vi "Invoke Specific Command.vi"(0 "LVx Command in":refnum<class "LVx.lvclass">, 5 "Session ID":string, 11 "error in (no error)":errorcluster) -> (4 "LVx Command out":refnum<class "LVx.lvclass">, 15 "error out":errorcluster)   [LabVIEW 2011, in "LVx.lvlib" / "LVx.lvclass"]
uses:
  LVx.lvclass
  LVx.lvclass/LVx.ctl
  LVx.lvlib
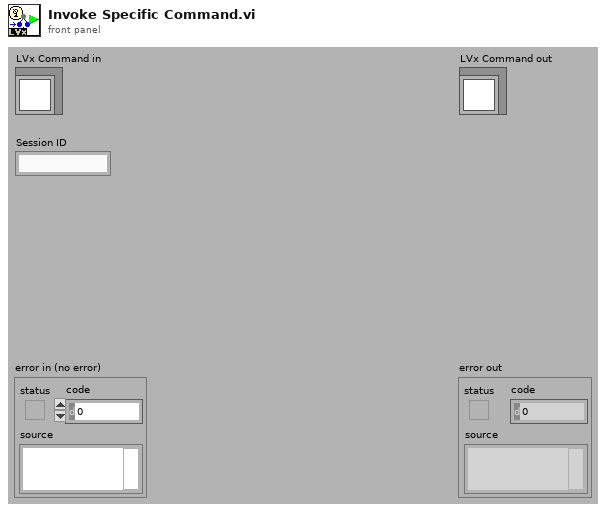
[diagram p1: front panel]
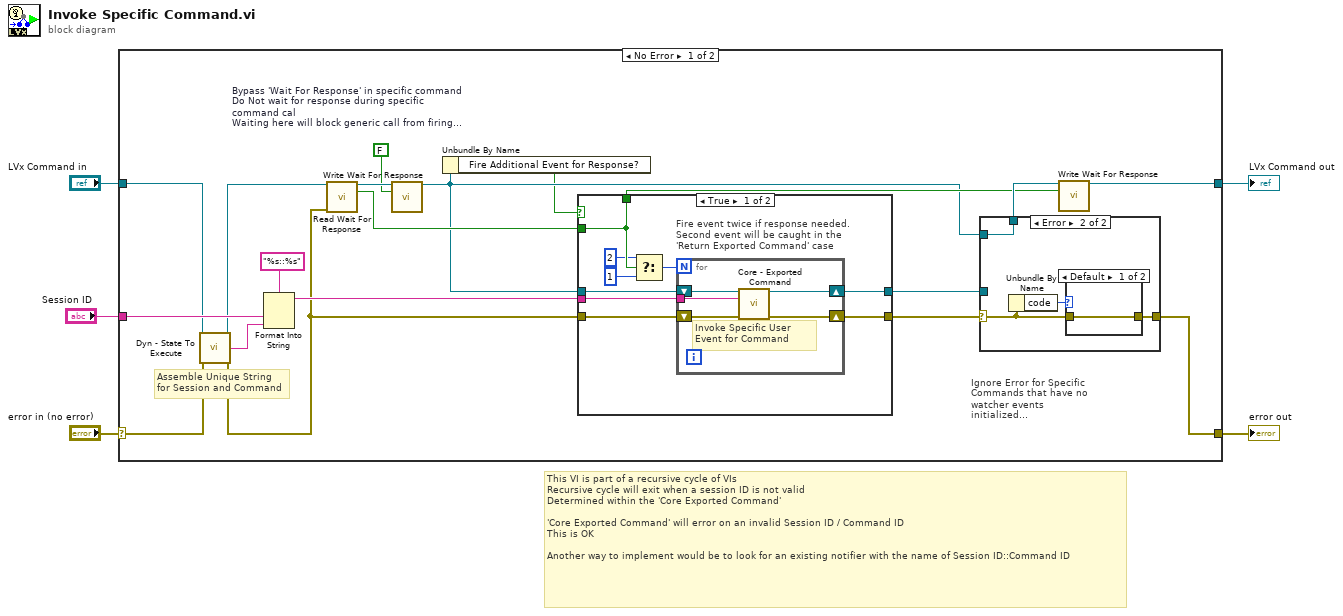
[diagram p0: block diagram]
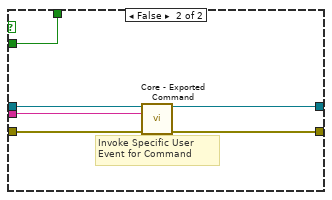
[diagram p2: hidden frame]
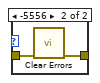
[diagram p4: hidden frame]
diagram:
  # "This VI is part of a recursive cycle of VIs\nRecursive cycle will exit when a session ID is not valid\nDetermined within the 'Core Exported Command'\n\n'Core Exported Command' will error on an invalid Session ID / Command ID\nThis is OK\n\nAnother way to implement would be to look for an existing notifier with the name of Session ID::Command ID"
  n1 = case shown="No Error" "error in (no error)" {
    selector: "error in (no error)" -> [w20 w55]
    tunnel: [w16 w55] -> w4
    tunnel: [w10 w54] -> w2
    tunnel: "LVx Command in" -> [w19 w54]
    tunnel: "Session ID" -> [w24 _]
    frame No Error {
      w12 = FALSE  # Bypass 'Wait For Response' in specific command Do Not wait for response during specific command cal Waiting here will block generic call from firing because of wait Response is caught in the calling VI (F)
      # "Assemble Unique String for Session and Command"
      n2 = call-dynamic "Dyn - State To Execute.vi"("LVx Command in"=w19, "error in (no error)"=w20) -> ("LVx Command out"=w15:refnum<class "LVx.lvclass">, "State To Execute"=w23:string, "error out"=w13:errorcluster)  [unwired: 11 in]
      n3 = Format Into String(format string="%s::%s", w24, w23) -> (resulting string=w21:string)  [unwired: 2 in, 1 out]
      n4 = call-dynamic "Read Wait For Response.vi"("LVx.lvclass in"=w15, "error in (no error)"=w13) -> ("LVx.lvclass out"=w14:refnum<class "LVx.lvclass">, "Wait For Response?"=w9:bool)  [unwired: 11 in, 1 out]
      n5 = call "Write Wait For Response.vi"("LVx.lvclass in"=w14, "Wait For Response? (T)"=w12) -> ("LVx.lvclass out"=w7:refnum<class "LVx.lvclass">)  [unwired: 12 in, 1 out]
      n6 = Unbundle By Name(w7) -> ("Fire Additional Event for Response?"=w6:bool)
      n7 = case shown="True" w6 {
        tunnel: w21 -> [w33 w44]
        tunnel: [w32 w43] -> w18
        tunnel: [w31 w42] -> w17
        tunnel: w13 -> [w30 w41]
        tunnel: w7 -> [w29 w40]
        tunnel: w9 -> [w28 w39]
        tunnel: [w28 w39] -> w8
        frame True {
          n8 = Select(t=2, s=w28, f=1) -> (s? t:f=w25:i32)
          n9 = for "Fire event twice if response needed.\nSecond event will be caught in the\n'Return Exported Command' case" {
            N: w25 -> [_]
            tunnel: w33 -> [w38]
            shift-right: [w36] -> w31
            shift-left: w29 -> [w34]
            shift-right: [w37] -> w32
            shift-left: w30 -> [w35]
            # "Invoke Specific User Event for Command"
            n10 = call "Core - Exported Command.vi"("LVx Command in"=w34, "Session ID"=w38, "error in (no error)"=w35) -> ("LVx Command out"=w36:refnum<class "LVx.lvclass">, "error out"=w37:errorcluster)  [unwired: 1 in, 10 out]
          }
        }
        frame False {
          # "Invoke Specific User Event for Command"
          n11 = call "Core - Exported Command.vi"("LVx Command in"=w40, "Session ID"=w44, "error in (no error)"=w41) -> ("LVx Command out"=w42:refnum<class "LVx.lvclass">, "error out"=w43:errorcluster)  [unwired: 1 in, 10 out]
        }
      }
      n12 = case "Ignore Error for Specific Commands that have no watcher events initialized\n\nMay need to find better solution for when user wants to know init did not happen" shown="Error" w18 {
        selector: w18 -> [w46 w48]
        tunnel: [w46 w49] -> w16
        tunnel: [w45 w47] -> w11
        tunnel: w17 -> [w45 _]
        tunnel: w7 -> [_ w47]
        frame No Error {
        }
        frame Error {
          n13 = Unbundle By Name(w48) -> ("code"=w50:i32)
          n14 = case shown="Default" w50 {
            tunnel: [w51 w53] -> w49
            tunnel: w48 -> [w51 w52]
            frame Default {
            }
            frame -5556 {
              n15 = call <vilib>:"Clear Errors.vi"("error in (no error)"=w52) -> ("error out"=w53:errorcluster)  [unwired: 6 in]
            }
          }
        }
      }
      n16 = call "Write Wait For Response.vi"("LVx.lvclass in"=w11, "Wait For Response? (T)"=w8) -> ("LVx.lvclass out"=w10:refnum<class "LVx.lvclass">)  [unwired: 12 in, 1 out]
    }
    frame Error {
    }
  }
  "error out" <- w4
  "LVx Command out" <- w2
